vi "Configure Sensor Location.vi"(6 "Sensor Location (0 meter)":dbl, 7 "Enable Auto Location (Enabled)":bool=TRUE, 8 "error in (no error)":errorcluster, 9 "Sensor Number (1)":i32=1, 10 "Channel (1: Channel 1)":i32(ring)=1 items=["All"=0, "Channel 1"=1, "Channel 1.1"=11, "Channel 1.2"=12, "Channel 1.3"=13, "Channel 1.4"=14, "Channel 2"=2, "Channel 2.1"=21, "Channel 2.2"=22, "Channel 2.3"=23, "Channel 2.4"=24, "Channel 3"=3, "Channel 3.1"=31, "Channel 3.2"=32, "Channel 3.3"=33, "Channel 3.4"=34, "Channel 4"=4, "Channel 4.1"=41, "Channel 4.2"=42, "Channel 4.3"=43, "Channel 4.4"=44], 11 "VISA resource name":refnum<visa-resource-name>) -> (0 "error out":errorcluster, 3 "VISA resource name out":refnum<visa-resource-name>)   [LabVIEW 2015, in "Micron Optics sm130.lvlib"]
doc: "Configures auto or manual sensor location to specified channel and sensor number. \nFor auto sensor location, this VI runs Measure Sensor Location.vi before applying the desired channel and sensor location. \nFor manual sensor location, user has to enter the sensor location in meters including the channel and sensor number."
uses:
  Micron Optics sm130.lvlib
panel:
  # "If Auto Location is enabled, Sensor Location control is ignored."
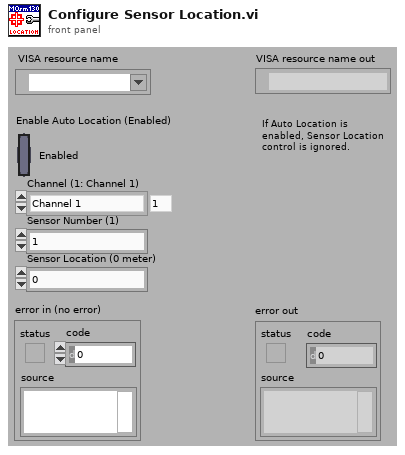
[diagram p1: front panel]
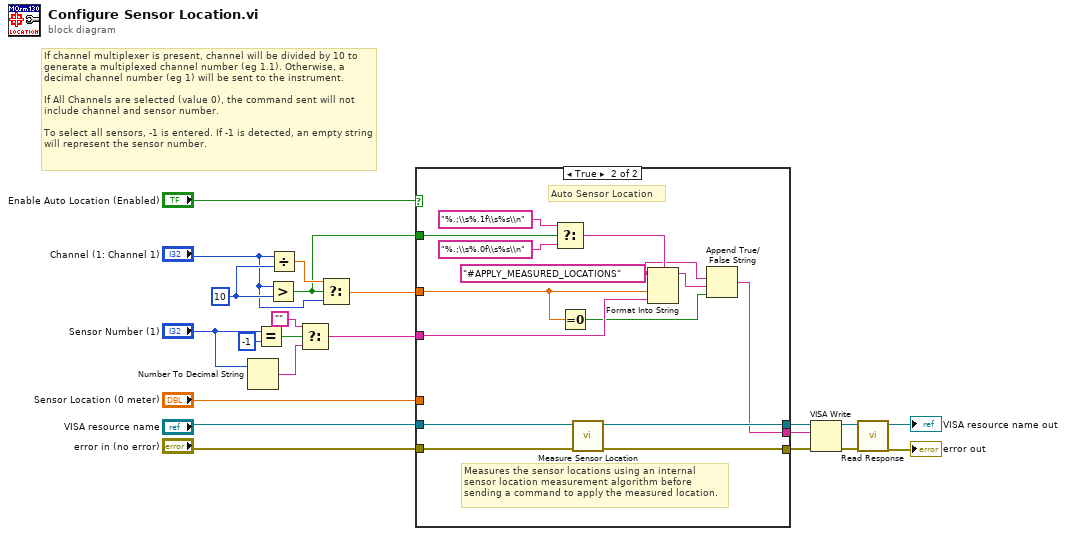
[diagram p0: block diagram]
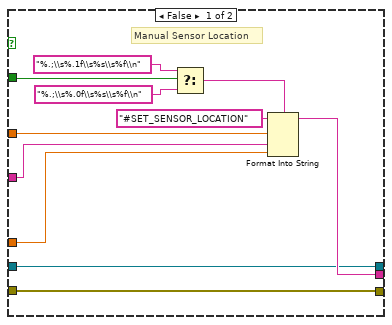
[diagram p2: hidden frame]
diagram:
  w19 = 10 ("y")
  # "If channel multiplexer is present, channel will be divided by 10 to generate a multiplexed channel number (eg 1.1). Otherwise, a decimal channel number (eg 1) will be sent to the instrument.\n\nIf All Channels are selected (value 0), the command sent will not include channel and sensor number. \n \nTo select all sensors, -1 is entered. If -1 is detected, an empty string will represent the sensor number."
  n1 = Number To Decimal String(number="Sensor Number (1)") -> (decimal integer string=w12:string)  [unwired: 1 in]
  n2 = Equal?(x="Sensor Number (1)", y=-1) -> (x = y?=w16:bool)
  n3 = Greater?(x="Channel (1: Channel 1)", y=w19) -> (0:w18:bool)
  n4 = Divide(x="Channel (1: Channel 1)", y=w19) -> (x/y=w20:dbl)
  n5 = Select(t="", s=w16, f=w12) -> (s? t:f=w14:string)
  n6 = Select(t=w20, s=w18, f="Channel (1: Channel 1)") -> (s? t:f=w13:dbl)
  n7 = case shown="True" "Enable Auto Location (Enabled)" {
    tunnel: "VISA resource name" -> [w24 w47]
    tunnel: "error in (no error)" -> [w23 w46]
    tunnel: w18 -> [w29 w45]
    tunnel: w14 -> [w27 w44]
    tunnel: w13 -> [w28 w40]
    tunnel: [w24 w36] -> w6
    tunnel: [w23 w35] -> w5
    tunnel: [w25 w34] -> w2
    tunnel: "Sensor Location (0 meter)" -> [w26 _]
    frame False {
      # "Manual Sensor Location"
      n8 = Select(t="%.;\\s%.1f\\s%s\\s%f\\n" ("format string"), s=w29, f="%.;\\s%.0f\\s%s\\s%f\\n" ("format string")) -> (s? t:f=w31:string)
      n9 = Format Into String(format string=w31, initial string="#SET_SENSOR_LOCATION", w28, w27, w26) -> (resulting string=w25:string)  [unwired: 1 in, 1 out]
    }
    frame True {
      w38 = "#APPLY_MEASURED_LOCATIONS" ("initial string")
      # "Auto Sensor Location"
      # "Measures the sensor locations using an internal sensor location measurement algorithm before sending a command to apply the measured location."
      n10 = Select(t="%.;\\s%.1f\\s%s\\n" ("format string"), s=w45, f="%.;\\s%.0f\\s%s\\n" ("format string")) -> (s? t:f=w41:string)
      n11 = Equal To 0?(x=w40) -> (x = 0?=w37:bool)
      n12 = call "Measure Sensor Location.vi"("error in (no error)"=w46, "VISA resource name"=w47) -> ("error out"=w35:errorcluster, "VISA resource name out"=w36:refnum<visa-resource-name>)  [unwired: 8 in]
      n13 = Format Into String(format string=w41, initial string=w38, w40, w44) -> (resulting string=w39:string)  [unwired: 1 in, 1 out]
      n14 = Append True/False String(1:w37, 2:w39, 3:w38) -> (0:w34:string)  [unwired: 1 in]
    }
  }
  n15 = VISA Write(VISA resource name=w6, write buffer=w2, error in (no error)=w5) -> (VISA resource name out=w7:refnum<visa-resource-name>, error out=w8:errorcluster)  [unwired: 1 out]
  n16 = call "Read Response.vi"("error in (no error)"=w8, "VISA resource name"=w7) -> ("error out"=→"error out":errorcluster, "VISA resource name out"=→"VISA resource name out":refnum<visa-resource-name>)  [unwired: 7 in, 1 out]
